vi "bracket code.vi"(11 "Enum":T1(ring)) -> (2 "Numeric":u8, 3 "Numeric 2":u8)   [LabVIEW 2017, in "API String Arguments Support.lvlib"]
uses:
  API String Arguments Support.lvlib
  <userlib>/_NEVSTOP/Communicable State Machine(CSM)/Communicable State Machine.lvlib
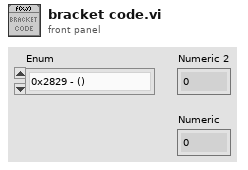
[diagram p1: front panel]
types:
  T1 = enum16{"0x2829 - ()", "0x5B5D - []", "0x7B7D - {}"}
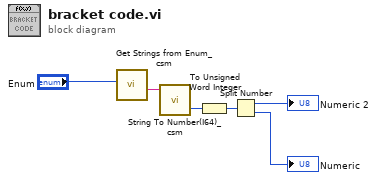
[diagram p0: block diagram]
diagram:
  n1 = call <userlib>:"Get Strings from Enum_csm.vi"("Enum"="Enum") -> ("String Value"=w2:string)  [unwired: 7 in, 3 out]
  n2 = call "String To Number(I64)_csm.vi"("String"=w2) -> ("Numeric(I64)"=w3:u64)  [unwired: 4 in]
  n3 = To Unsigned Word Integer(number=w3) -> (unsigned 16bit integer=w4:u16)
  n4 = Split Number(x=w4) -> (hi(x)=→"Numeric 2":u8, lo(x)=→"Numeric":u8)
